vi "run.free.vi"(8 "error in":errorcluster, 11 "Run in":refnum<class "Run.lvclass">) -> (0 "error out":errorcluster, 3 "Run out":refnum<class "Run.lvclass">)   [LabVIEW 2020, in "Run.lvclass"]
doc: "Releases the handle and its associated resources."
uses:
  Run.lvclass
  Run.lvclass/Run.ctl
  client.lvlib
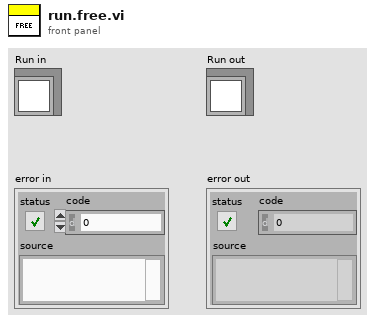
[diagram p1: front panel]
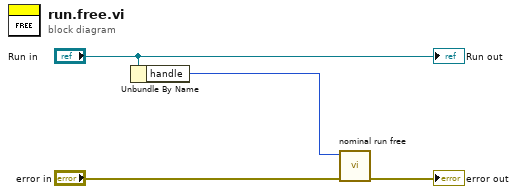
[diagram p0: block diagram]
diagram:
  n1 = Unbundle By Name("Run in") -> ("handle"=w2:i32)
  n2 = call "nominal run free.vi"("error in (no error)"="error in", "run"=w2) -> ("error out"=→"error out":errorcluster)  [unwired: 8 in, 1 out]
  "Run out" <- "Run in"
